vi "Setup subWorker - Acq Cam.vi"(8 "error in":errorcluster, 11 "UI Cam Basler in":refnum<class "UI Cam Basler.lvclass">) -> (0 "error out":errorcluster, 3 "UI Cam Basler out":refnum<class "UI Cam Basler.lvclass">)   [LabVIEW 2023, in "UI Cam Basler.lvclass"]
doc: "<b>Note: Do not change the code in this VI!</b>\nThis VI performs a setup of all the statically-linked subWorkers that belong to the Worker that calls this VI. This VI is created automatically by the 'Create/Add Worker' tool and must be called <b>before</b> any statically linked subWorkers are called."
uses:
  UI Cam Basler.lvclass
  UI Cam Basler.lvclass/UI Cam Basler.ctl
  Acq Cam Basler/Acq Cam Basler.lvclass
  C:/Program Files (x86)/National Instruments/LabVIEW 2023/vi.lib/addons/_Workers/Library/Classes/Worker/Worker.lvclass
  C:/Program Files (x86)/National Instruments/LabVIEW 2023/vi.lib/addons/_Workers/Library/Classes/Workers Object/Workers Object.lvclass
  C:/Users/Fab/Contacts/Desktop/MDI-with-Labview-Workers/Workers/Acq Cam Basler/Acq Cam Basler.lvclass
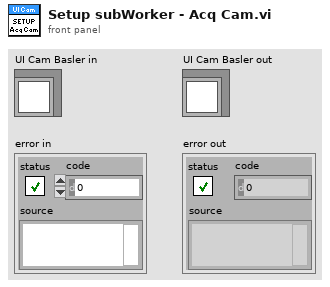
[diagram p1: front panel]
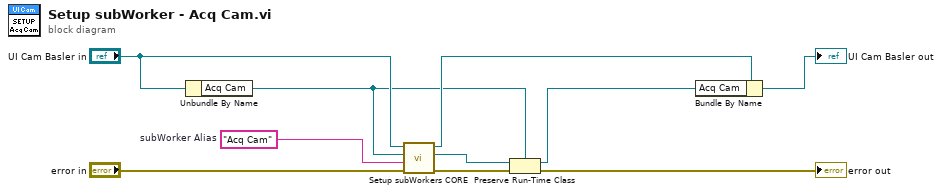
[diagram p0: block diagram]
diagram:
  w6 = "Acq Cam"  # subWorker Alias
  n1 = Unbundle By Name("UI Cam Basler in") -> ("Acq Cam"=w3:refnum<class "Acq Cam Basler.lvclass">)
  n2 = call-dynamic "Setup subWorkers CORE.vi"("error in"="error in", "subWorker Alias"=w6, "subWorker"=w3, "Worker"="UI Cam Basler in") -> ("error out"=w5:errorcluster, "subWorker out"=w1:refnum<class "Worker.lvclass">, "Worker out"=w8:refnum<class "UI Cam Basler.lvclass">)  [unwired: 5 in]
  n3 = Preserve Run-Time Class(object in=w1, error in=w5, 2:w3) -> (object out=w2:refnum<class "Acq Cam Basler.lvclass">, error out=→"error out":errorcluster)
  n4 = Bundle By Name(cluster=w8, "Acq Cam"=w2) -> (→"UI Cam Basler out":refnum<class "UI Cam Basler.lvclass">)
